vi "Result Data Update the Self.vi"(8 "error in (no error)":errorcluster, 10 "Report Data":T1={"Schema"="", "Test Socket"="", "Start Test Cycle"="", "Stop Test Cycle"="", "Test Mode"="", "Frame Type"="fe_frame_log"}, 11 "Import Export in":refnum<class "Import Export SQL.lvclass">) -> (0 "error out":errorcluster, 3 "Import Export out":refnum<class "Import Export SQL.lvclass">)   [LabVIEW 2023, in "Data Analysis.lvlib" / "Import Export SQL.lvlib" / "Import Export SQL.lvclass"]
uses:
  Import Export SQL.lvclass
  Control/Report.ctl
  Import Export SQL.lvclass/Import Export SQL.ctl
  Data Analysis.lvlib
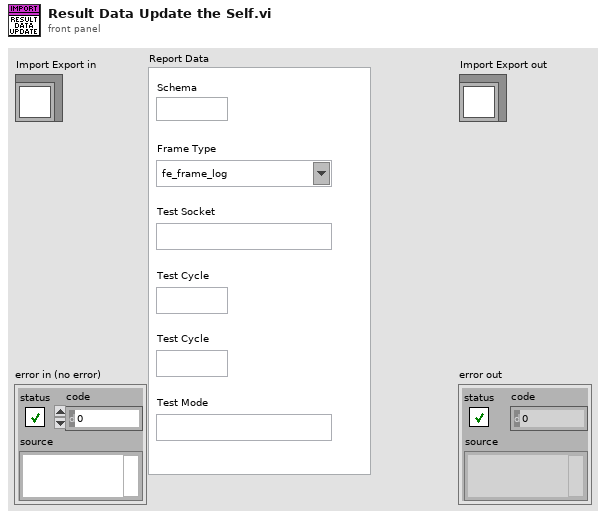
[diagram p1: front panel]
types:
  T1 = typedef "Data Analysis.lvlib/Report.ctl" = cluster{"Schema":string, "Test Socket":string, "Start Test Cycle":string, "Stop Test Cycle":string, "Test Mode":string, "Frame Type":string}
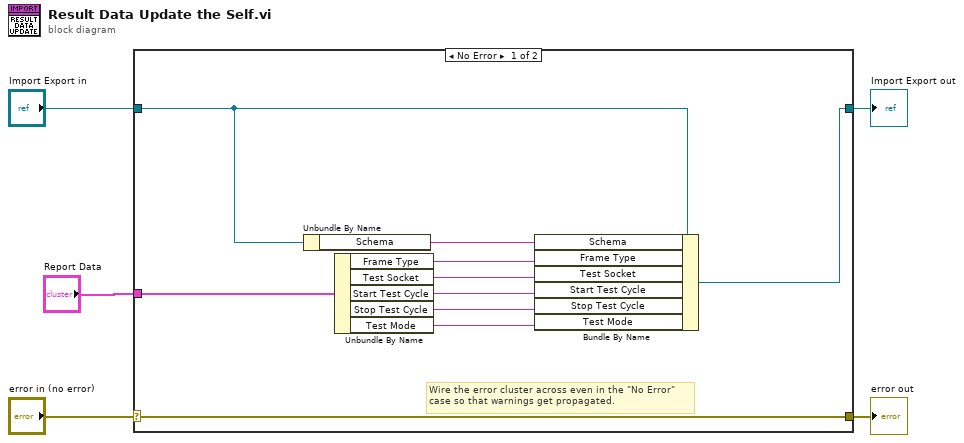
[diagram p0: block diagram]
diagram:
  n1 = case shown="No Error" "error in (no error)" {
    selector: "error in (no error)" -> [w15 w17]
    tunnel: [w15 w17] -> w4
    tunnel: [w8 w16] -> w2
    tunnel: "Import Export in" -> [w6 w16]
    tunnel: "Report Data" -> [w7 _]
    frame No Error {
      # "Wire the error cluster across even in the \"No Error\"\ncase so that warnings get propagated."
      n2 = Unbundle By Name(w6) -> ("Schema"=w14:string)
      n3 = Unbundle By Name(w7) -> ("Frame Type"=w13:string, "Test Socket"=w12:string, "Start Test Cycle"=w11:string, "Stop Test Cycle"=w10:string, "Test Mode"=w9:string)
      n4 = Bundle By Name(cluster=w6, "Schema"=w14, "Frame Type"=w13, "Test Socket"=w12, "Start Test Cycle"=w11, "Stop Test Cycle"=w10, "Test Mode"=w9) -> (w8:refnum<class "Import Export SQL.lvclass">)
    }
    frame Error {
    }
  }
  "error out" <- w4
  "Import Export out" <- w2
